vi "PinholesSingle.vi"(4 "Current Threshold [nA]":dbl, 6 "Channel":i32) -> (0 "Compliance?":bool, 1 "channel excluded":bool, 2 "Current [nA]":dbl, 3 "Flag":i32)   [LabVIEW 2013]
uses:
  InstrControl/Switching/Switching.lvclass
  InstrControl/SupplyControl/SupplyControl.lvclass
  general_VIs/globals/QC_MeasurementSetup.vi
panel:
  in  "settling\ndelay":i32
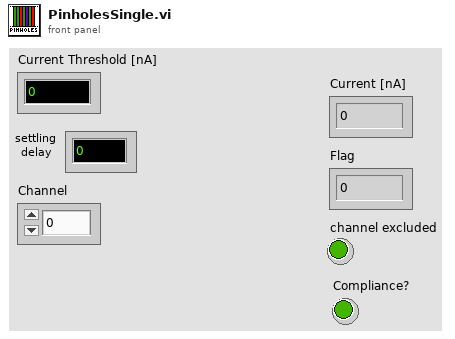
[diagram p1: front panel]
types:
  T1 = cluster{"Bias Supply":refnum<class "SupplyControl.lvclass">, "SMU":refnum<class "SupplyControl.lvclass">, "LCR":refnum<class "LCRControl.lvclass">, "Probe Card Channels":i32, "Bias Voltage [V]":dbl, "First strip":i32, "Last strip":i32, "Base Voltage [V]":dbl, "Base Ramp Step [V]":dbl, "Base Ramp Interval [ms]":u32, "High Voltage [V]":dbl, "High Ramp Step [V]":dbl, "High Ramp Interval [ms]":u32, "Single Needle":bool, "Temperature Readout":enum16{"Read Arduino", "Enter manually"}, "Arduino":refnum<class "ArduinoControl.lvclass">, "Fraction of good strips [%]":dbl, "ProbeStation":refnum<class "ProbeStationControl.lvclass">, "AC frequency [Hz]":i32, "Switching":refnum<class "Switching.lvclass">, "Matrix used?":bool, "Matrix X Channels":cluster{"Bias Supply / SMU LO":i32, "Bias Supply / SMU HI":i32, "CV Box LO":i32, "CV Box HI":i32, "CV Box LO IN":i32, "CV Box HI IN":i32, "Volt meter LO":i32, "Volt meter HI":i32, "Mux1 C1":i32, "Mux1 C2":i32, "Mux2 C1":i32, "Mux2 C2":i32}, "Pinholes Y/N":bool, "Capacitance Y/N":bool, "Resistance Y/N":bool}
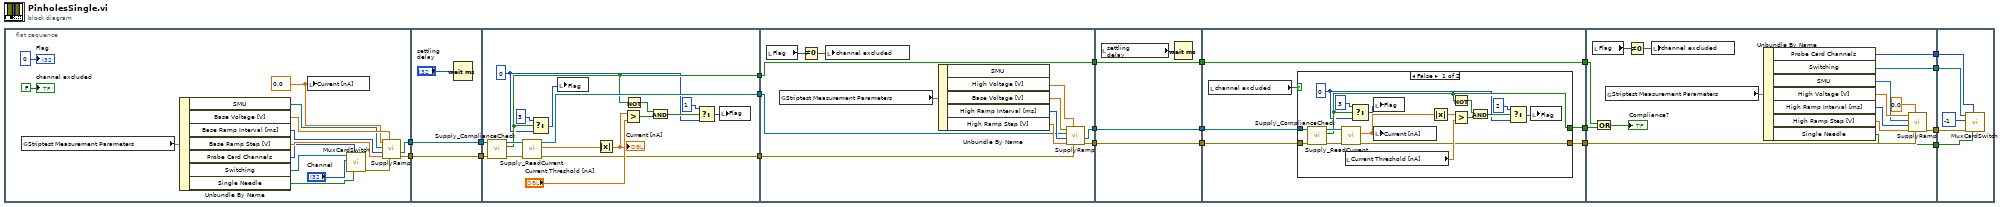
[diagram p0: block diagram]
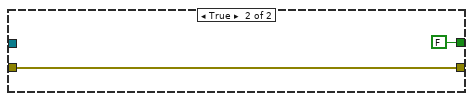
[diagram p2: hidden frame]
diagram:
  n1 = flat-sequence {
    tunnel: [w27] -> w14
    tunnel: [w26] -> w12
    tunnel: [w37] -> w15
    tunnel: w14 -> [w37]
    tunnel: [w36] -> w13
    tunnel: w12 -> [w36]
    tunnel: [w45] -> w20
    tunnel: w15 -> [w49]
    tunnel: w13 -> [w48]
    tunnel: [w47] -> w11
    tunnel: [w46] -> w10
    tunnel: w20 -> [w68]
    tunnel: [w68] -> w17
    tunnel: w11 -> [w62]
    tunnel: w10 -> [w61]
    tunnel: [w60] -> w8
    tunnel: [w59] -> w4
    tunnel: w17 -> [w72]
    tunnel: [w72] -> w16
    tunnel: [w70] -> w9
    tunnel: w8 -> [w70]
    tunnel: [w69] -> w5
    tunnel: w4 -> [w69]
    tunnel: w16 -> [w78]
    tunnel: [w78] -> w19
    tunnel: [w77] -> w18
    tunnel: w9 -> [w75]
    tunnel: [w74] -> w7
    tunnel: w5 -> [w73]
    tunnel: w19 -> [w102]
    tunnel: w18 -> [w101]
    tunnel: w7 -> [w107]
    tunnel: [w106] -> w6
    tunnel: [w100] -> w3
    tunnel: [w99] -> w2
    tunnel: [w98] -> w1
    tunnel: w6 -> [w117]
    tunnel: w3 -> [w116]
    tunnel: w2 -> [w115]
    tunnel: w1 -> [w114]
    frame #0 {
      w29 = 0.0 ("Starting Voltage")
      n2 = global read "QC_MeasurementSetup.vi" "Striptest Measurement Parameters"() -> (w30:T1)
      n3 = Unbundle By Name(w30) -> ("SMU"=w25:refnum<class "SupplyControl.lvclass">, "Base Voltage [V]"=w31:dbl, "Base Ramp Interval [ms]"=w32:u32, "Base Ramp Step [V]"=w33:dbl, "Probe Card Channels"=w21:i32, "Switching"=w22:refnum<class "Switching.lvclass">, "Single Needle"=w23:bool)
      n4 = local write "Current [nA]"(w29) -> ()
      n5 = call-dynamic "MuxCardSwitch.vi"("Single Needle"=w23, "Probe Card Channels"=w21, "Switch to channel"="Channel", "Switching in"=w22) -> ("error out"=w28:errorcluster)  [unwired: 5 in, 2 out]
      n6 = call "SupplyRamp.vi"("error in"=w28, "Requested Voltage"=w31, "Step Size"=w33, "Step Delay"=w32, "Supply IN"=w25, "Starting Voltage"=w29) -> ("error out"=w27:errorcluster, "Supply OUT"=w26:refnum<class "SupplyControl.lvclass">)  [unwired: 2 in, 2 out]
      "Flag" <- 0
      "channel excluded" <- FALSE
    }
    frame #1 {
      n7 = Wait (ms)(milliseconds to wait="settling\ndelay") -> ()  [unwired: 1 out]
    }
    frame #2 {
      w39 = 0
      n8 = call-dynamic "Supply_ComplianceCheck.vi"("error in (no error)"=w49, "SupplyControl in"=w48) -> ("error out"=w51:errorcluster, "Compliance exceeded?"=w45:bool, "SupplyControl out"=w52:refnum<class "SupplyControl.lvclass">)  [unwired: 6 in, 1 out]
      n9 = call-dynamic "Supply_ReadCurrent.vi"("error in (no error)"=w51, "SupplyControl in"=w52) -> ("error out"=w46:errorcluster, "Current in nA"=w56:dbl, "SupplyControl out"=w47:refnum<class "SupplyControl.lvclass">)  [unwired: 7 in]
      n10 = Select(t=3, s=w45, f=w39) -> (s? t:f=w44:i32)
      n11 = local write "Flag"(w44) -> ()
      n12 = Absolute Value(x=w56) -> (abs(x)=w50:dbl)
      "Current [nA]" <- w50
      n13 = Greater?(x=w50, y="Current Threshold [nA]") -> (0:w53:bool)
      n14 = Not(x=w45) -> (.not. x?=w54:bool)
      n15 = And(x=w54, y=w53) -> (x .and. y?=w42:bool)
      n16 = Select(t=1, s=w42, f=w39) -> (s? t:f=w41:i32)
      n17 = local write "Flag"(w41) -> ()
    }
    frame #3 {
      n18 = local read "Flag"() -> (w57:i32)
      n19 = global read "QC_MeasurementSetup.vi" "Striptest Measurement Parameters"() -> (w64:T1)
      n20 = Not Equal To 0?(x=w57) -> (x != 0?=w58:bool)
      n21 = local write "channel excluded"(w58) -> ()
      n22 = Unbundle By Name(w64) -> ("High Voltage [V]"=w63:dbl, "Base Voltage [V]"=w67:dbl, "High Ramp Interval [ms]"=w66:u32, "High Ramp Step [V]"=w65:dbl)  [unwired: 1 out]
      n23 = call "SupplyRamp.vi"("error in"=w61, "Requested Voltage"=w63, "Step Size"=w65, "Step Delay"=w66, "Supply IN"=w62, "Starting Voltage"=w67) -> ("error out"=w60:errorcluster, "Supply OUT"=w59:refnum<class "SupplyControl.lvclass">)  [unwired: 2 in, 2 out]
    }
    frame #4 {
      n24 = local read "settling\ndelay"() -> (w71:i32)
      n25 = Wait (ms)(milliseconds to wait=w71) -> ()  [unwired: 1 out]
    }
    frame #5 {
      n26 = local read "channel excluded"() -> (w76:bool)
      n27 = case shown="False" w76 {
        tunnel: [w80 FALSE] -> w77
        tunnel: w75 -> [w88 w96]
        tunnel: [w87 w96] -> w74
        tunnel: w73 -> [w86 _]
        frame False {
          w79 = 0
          n28 = call-dynamic "Supply_ComplianceCheck.vi"("error in (no error)"=w88, "SupplyControl in"=w86) -> ("error out"=w89:errorcluster, "Compliance exceeded?"=w80:bool, "SupplyControl out"=w90:refnum<class "SupplyControl.lvclass">)  [unwired: 6 in, 1 out]
          n29 = call-dynamic "Supply_ReadCurrent.vi"("error in (no error)"=w89, "SupplyControl in"=w90) -> ("error out"=w87:errorcluster, "Current in nA"=w95:dbl)  [unwired: 7 in, 1 out]
          n30 = local read "Current Threshold [nA]"() -> (w92:dbl)
          n31 = Select(t=3, s=w80, f=w79) -> (s? t:f=w83:i32)
          n32 = local write "Flag"(w83) -> ()
          n33 = local write "Current [nA]"(w95) -> ()
          n34 = Absolute Value(x=w95) -> (abs(x)=w91:dbl)
          n35 = Not(x=w80) -> (.not. x?=w94:bool)
          n36 = Greater?(x=w91, y=w92) -> (0:w93:bool)
          n37 = And(x=w94, y=w93) -> (x .and. y?=w81:bool)
          n38 = Select(t=2, s=w81, f=w79) -> (s? t:f=w82:i32)
          n39 = local write "Flag"(w82) -> ()
        }
        frame True {
        }
      }
    }
    frame #6 {
      n40 = local read "Flag"() -> (w104:i32)
      n41 = Or(x=w102, y=w101) -> (x .or. y?=→"Compliance?":bool)
      n42 = global read "QC_MeasurementSetup.vi" "Striptest Measurement Parameters"() -> (w109:T1)
      n43 = Not Equal To 0?(x=w104) -> (x != 0?=w105:bool)
      n44 = local write "channel excluded"(w105) -> ()
      n45 = Unbundle By Name(w109) -> ("Probe Card Channels"=w99:i32, "Switching"=w100:refnum<class "Switching.lvclass">, "SMU"=w110:refnum<class "SupplyControl.lvclass">, "High Voltage [V]"=w113:dbl, "High Ramp Interval [ms]"=w112:u32, "High Ramp Step [V]"=w111:dbl, "Single Needle"=w98:bool)
      n46 = call "SupplyRamp.vi"("error in"=w107, "Requested Voltage"=0.0, "Step Size"=w111, "Step Delay"=w112, "Supply IN"=w110, "Starting Voltage"=w113) -> ("error out"=w106:errorcluster)  [unwired: 2 in, 3 out]
    }
    frame #7 {
      n47 = call-dynamic "MuxCardSwitch.vi"("Single Needle"=w114, "Probe Card Channels"=w115, "error in (no error)"=w117, "Switch to channel"=-1, "Switching in"=w116) -> ()  [unwired: 4 in, 3 out]
    }
  }
